vi "Handle Error.vi"(8 "error in (no error)":errorcluster, 11 "Child_1 in":refnum<class "Child_2_Class.lvclass">=refnum) -> (0 "error out":errorcluster, 2 "stop actor?":bool=TRUE, 3 "Child_1 out":refnum<class "Child_2_Class.lvclass">)   [LabVIEW 2023, in "Actor_Child_2.lvlib" / "Child_2_Class.lvclass"]
doc: "(<B>Filename</B>: Actor Framework.lvlib:Actor.lvclass:Handle Error.vi)\n\nDefines how the actor handles an error that occurred while processing a message. By default, this method does nothing except stop the actor."
uses:
  Child_2_Class.lvclass
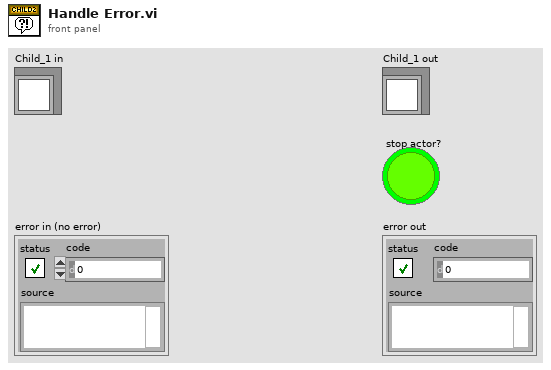
[diagram p1: front panel]
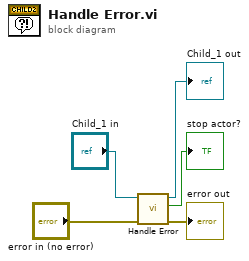
[diagram p0: block diagram]
diagram:
  n1 = call-parent "Handle Error.vi"("error in (no error)"="error in (no error)", "Actor in"="Child_1 in") -> ("error out"=→"error out":errorcluster, "stop actor?"=→"stop actor?":bool, "Actor out"=→"Child_1 out":refnum<class "Child_2_Class.lvclass">)  [unwired: 7 in]
